vi "Get Double.vi"(7 "data type of variable":dbl, 8 "error in":errorcluster, 10 "variable name":string, 11 "GOLPI ref. in":T1={"pipe handle"={"lv_proc.dll file path"=path "", "process instance handle"=[], "debug mode"=FALSE, "debug data"=[]}, "fast read timeout [ms]"=500, "fast read settle time [ms]"=10, "fast read to multiple [ms]"=1, "max elements per input line"=100, "slow read timeout [ms]"=5000, "stdin double format specifier"="%_16e", "max elements per stdout output column"=100}) -> (0 "error out":errorcluster, 2 "value":dbl format="%.2f", 3 "GOLPI ref. out":T1={"pipe handle"={"lv_proc.dll file path"=path "", "process instance handle"=[], "debug mode"=FALSE, "debug data"=[]}, "fast read timeout [ms]"=500, "fast read settle time [ms]"=10, "fast read to multiple [ms]"=1, "max elements per input line"=100, "slow read timeout [ms]"=5000, "stdin double format specifier"="%_16e", "max elements per stdout output column"=100})   [LabVIEW 2013, in "GOLPI library.lvlib"]
doc: "Part of polymorph Get Variable.vi"
uses:
  GOLPI library.lvlib
  Public/GOLPI reference Type Def.ctl
  LV Process source distribution/Pipe Handle.ctl
  Type Definitions/Custom Error Codes Enum Type Def.vi
  LV Process source distribution/LV Process library.lvlib
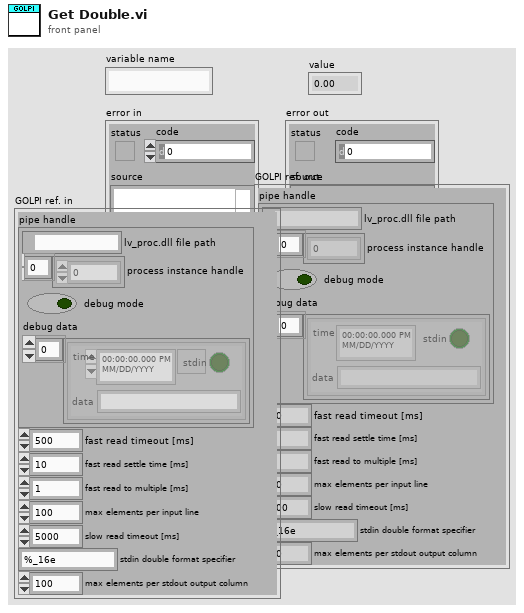
[diagram p1: front panel]
types:
  T1 = typedef "GOLPI library.lvlib/GOLPI reference Type Def.ctl" = cluster{"pipe handle":T2, "fast read timeout [ms]":u32, "fast read settle time [ms]":u32, "fast read to multiple [ms]":u32, "max elements per input line":u32, "slow read timeout [ms]":u32, "stdin double format specifier":string, "max elements per stdout output column":u32}
  T2 = typedef "LV Process library.lvlib/Pipe Handle.ctl" = cluster{"lv_proc.dll file path":path, "process instance handle":u32[], "debug mode":bool, "debug data":cluster{"time":timestamp, "stdin":bool, "data":string}[]}
  T3 = typedef "GOLPI library.lvlib/Custom Error Codes Enum Type Def.vi" = enum16{"no error", "00 working directory PAR1 missing", "01 octave binary PAR1 missing", "02 octave report error PAR1", "03 empty output last cmd PAR1", "04 missing temporary file PAR1", "05 pwd PAR 1 not exist", "10 var PAR1 not string, vect", "11 var PAR1 not num, scal, ~compl", "12 var PAR1 not num, scal, compl", "13 var PAR1 not num, vect, ~compl", "14 var PAR1 not num, vect, compl", "15 var PAR1 not num, mat, ~compl", "16 var PAR1 not num, mat, ~compl", "30 read timeout", "99 not finished"}
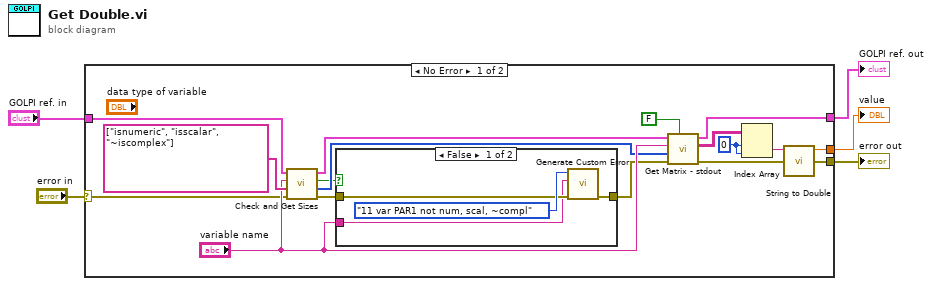
[diagram p0: block diagram]
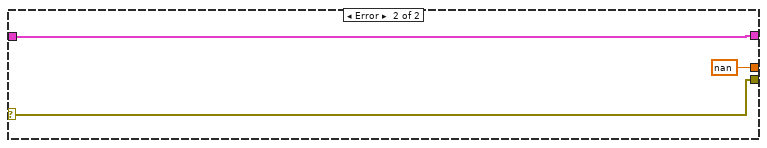
[diagram p3: hidden frame]
diagram:
  n1 = case shown="No Error" "error in" {
    selector: "error in" -> [w11 w29]
    tunnel: [w6 nan ("t")] -> w5
    tunnel: [w8 w29] -> w4
    tunnel: "GOLPI ref. in" -> [w14 w27]
    tunnel: [w12 w27] -> w1
    frame No Error {
      w15 = 0 ("index (row)")
      n2 = call "Check and Get Sizes.vi"("error in (no error)"=w11, "test commands"=string[] ["isnumeric", "isscalar", "~iscomplex"], "variable name"="variable name", "GOLPI ref. in"=w14) -> ("error out"=w10:errorcluster, "octave sizes"=w19:i32[], "all tests OK?"=w18:bool, "GOLPI ref. out"=w13:T1)  [unwired: 4 in]
      n3 = case shown="False" w18 {
        tunnel: [w23 w26] -> w9
        tunnel: w10 -> [w24 w26]
        tunnel: "variable name" -> [w22 _]
        frame False {
          n4 = call "Generate Custom Error.vi"("error in"=w24, "PAR1"=w22, "GOLPI error"=Custom_Error_Codes_Enum_Type_Def.vi."11 var PAR1 not num, scal, ~compl" ("Enum")) -> ("error out"=w23:errorcluster)  [unwired: 8 in]
        }
        frame True {
        }
      }
      n5 = call "Get Matrix - stdout.vi"("is string?"=FALSE ("is string"), "error in (no error)"=w9, "octave sizes"=w19, "variable name"="variable name", "GOLPI ref. in"=w13) -> ("error out"=w8:errorcluster, "array"=w16:string[][], "GOLPI ref. out"=w12:T1)  [unwired: 4 in]
      n6 = Index Array(array=w16, index (row)=w15, index (col)=w15) -> (element=w7:string)
      n7 = call "String to Double.vi"("string"=w7) -> ("number"=w6:dbl)  [unwired: 10 in]
    }
    frame Error {
    }
  }
  "value" <- w5
  "error out" <- w4
  "GOLPI ref. out" <- w1
